vi "stop.vi"(8 "error in (no error)":errorcluster, 11 "Model in":refnum<class "Model.lvclass">) -> (0 "error out":errorcluster, 3 "Model out":refnum<class "Model.lvclass">)   [LabVIEW 2013, in "Model.lvclass"]
uses:
  Model.lvclass
  Model.lvclass/Model.ctl
  <userlib>/Common/ILC/ILC/ILC.lvclass
  <userlib>/Common/Devices/EncoderReader/EncoderReader/EncoderReader.lvclass
  <userlib>/Common/Devices/DistanceGauge/DistanceGauge/DistanceGauge.lvclass
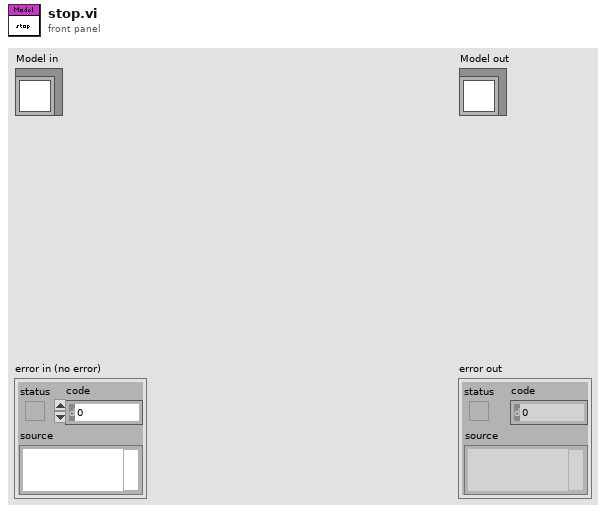
[diagram p1: front panel]
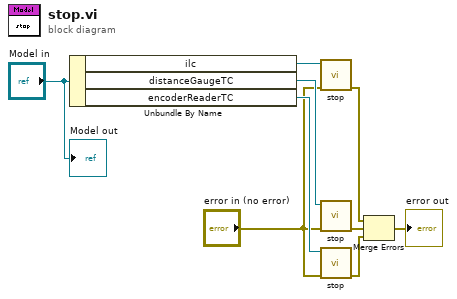
[diagram p0: block diagram]
diagram:
  n1 = Unbundle By Name("Model in") -> ("ilc"=w8:refnum<class "ILC.lvclass">, "distanceGaugeTC"=w7:refnum<class "DistanceGaugeTC.lvclass">, "encoderReaderTC"=w6:refnum<class "EncoderReaderTC.lvclass">)
  n2 = call <userlib>:"stop.vi"("error in (no error)"="error in (no error)", "ILC in"=w8) -> ("error out"=w4:errorcluster)  [unwired: 8 in, 1 out]
  n3 = call <userlib>:"stop.vi"("error in (no error)"="error in (no error)", "DistanceGauge in"=w7) -> ("error out"=w3:errorcluster)  [unwired: 8 in, 1 out]
  n4 = call <userlib>:"stop.vi"("error in (no error)"="error in (no error)", "EncoderReader in"=w6) -> ("error out"=w2:errorcluster)  [unwired: 8 in, 1 out]
  n5 = Merge Errors(w4, w3, w2) -> (→"error out":errorcluster)
  "Model out" <- "Model in"
